vi "niRFUtil WFM Pad Waveform (real wfm).vi"(0 "Waveform In":T2 {"y" min=0 max=127 format="%.2f"; "dx" format="%^.2e"; "x0" format="%^.2e"}, 2 "Padding Type (Zero)":T1(ring), 13 "Duration":dbl format="%^.2e") -> (4 "Waveform Out":T2 {"y" min=0 max=127 format="%.2f"; "dx" format="%^.2e"; "x0" format="%^.2e"})   [LabVIEW 2015, in "niRFUtil.lvlib"]
doc: "(c) Copyright 2006, National Instruments, Inc. This VI may not be duplicated, sold, or distributed without written consent from National Instruments."
uses:
  niRFUtil.lvlib
  Includes/niRFUtil INC Real Waveform.ctl
  Includes/niRFUtil INC Real Array.ctl
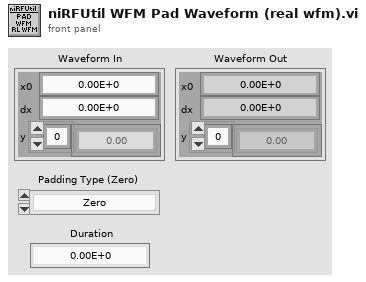
[diagram p1: front panel]
types:
  T1 = enum16{"Zero", "Leading/Trailing", "Cyclic Prefix/Postfix"}
  T2 = typedef "niRFUtil.lvlib/niRFUtil INC Real Waveform.ctl" = cluster{"x0":dbl, "dx":dbl, "y":T3}
  T3 = typedef "niRFUtil.lvlib/niRFUtil INC Real Array.ctl" = sgl[]
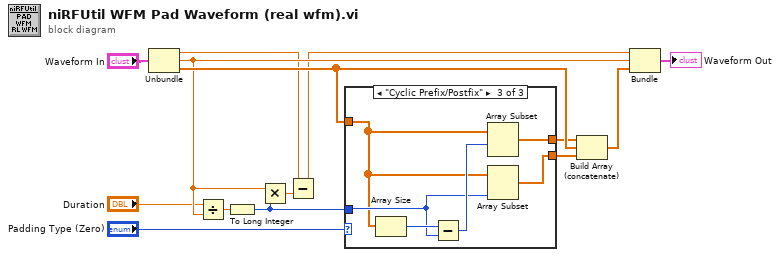
[diagram p0: block diagram]
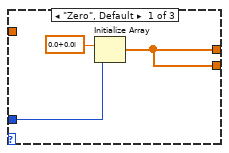
[diagram p2: hidden frame]
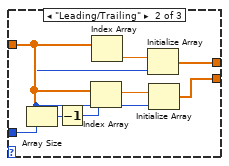
[diagram p3: hidden frame]
diagram:
  n1 = Unbundle("Waveform In") -> ("x0"=w6:dbl, "dx"=w8:dbl, "y"=w11:T3)
  n2 = Divide(x="Duration", y=w8) -> (x/y=w14:dbl)
  n3 = To Long Integer(number=w14) -> (32bit integer=w9:i32)
  n4 = Multiply(x=w8, y=w9) -> (x*y=w7:dbl)
  n5 = Subtract(x=w6, y=w7) -> (x-y=w5:dbl)
  n6 = case shown="\"Cyclic Prefix/Postfix\"" "Padding Type (Zero)" {
    tunnel: w9 -> [w15 w18 w29]
    tunnel: [w16 w19 w27] -> w12
    tunnel: w11 -> [_ w20 w28]
    tunnel: [w16 w24 w26] -> w10
    frame "Zero", Default {
      n7 = Initialize Array(csg 0.0+0.0i ("element"), w15) -> (w16:csg[])
    }
    frame "Leading/Trailing" {
      n8 = Array Size(array=w20) -> (size(s)=w22:i32)
      n9 = Decrement(x=w22) -> (x-1=w21:i32)
      n10 = Index Array(array=w20, index=w21) -> (element=w23:sgl)
      n11 = Index Array(array=w20) -> (element=w25:sgl)  [unwired: 1 in]
      n12 = Initialize Array(w25, w18) -> (w24:sgl[])
      n13 = Initialize Array(w23, w18) -> (w19:sgl[])
    }
    frame "Cyclic Prefix/Postfix" {
      n14 = Array Size(array=w28) -> (size(s)=w31:i32)
      n15 = Subtract(x=w31, y=w29) -> (x-y=w30:i32)
      n16 = Array Subset(array=w28, index=w30) -> (w26:T3)  [unwired: 1 in]
      n17 = Array Subset(array=w28, length=w29) -> (w27:T3)  [unwired: 1 in]
    }
  }
  n18 = Build Array (concatenate)(w10, w11, w12) -> (w13:csg[])
  n19 = Bundle(w5, "dx"=w8, w13) -> (→"Waveform Out":cluster{dbl, "dx":dbl, csg[]})  [unwired: 1 out]
